vi "_Read.vi"(8 "error in (no error)":errorcluster, 11 "Wavelength Meter in":refnum<class "Wavelength Meter.lvclass">) -> (0 "error out":errorcluster, 2 "4 Data Points":dbl[](array[numeric]), 3 "Wavelength Meter out":refnum<class "Wavelength Meter.lvclass">)   [LabVIEW 2023, in "Wavelength Meter.lvclass"]
uses:
  Wavelength Meter.lvclass
  Wavelength Meter.lvclass/Wavelength Meter.ctl
  Utility Classes/Readable/Readable.lvclass
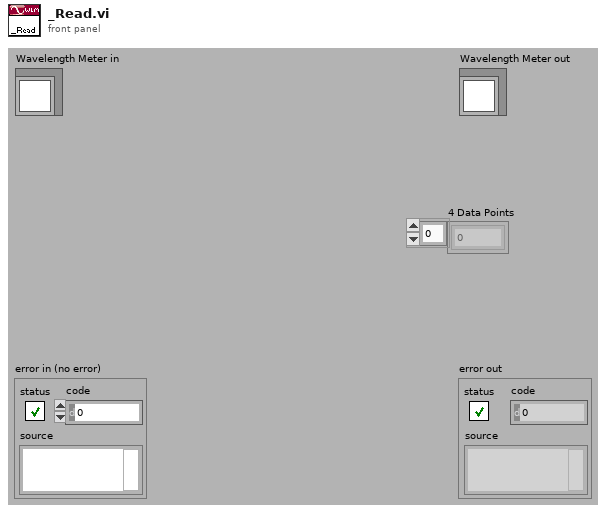
[diagram p1: front panel]
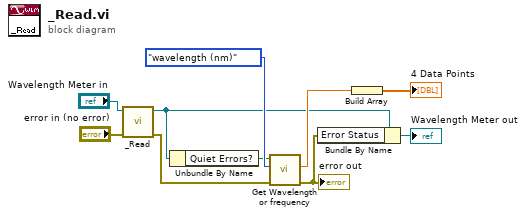
[diagram p0: block diagram]
diagram:
  n1 = call-parent "_Read.vi"("error in (no error)"="error in (no error)", "Readable in"="Wavelength Meter in") -> ("error out"=w5:errorcluster, "Readable out"=w4:refnum<class "Wavelength Meter.lvclass">)  [unwired: 8 out]
  n2 = Unbundle By Name(w4) -> ("Quiet Errors?"=w2:bool)
  n3 = call "Get Wavelength or frequency.vi"("error in (no error)"=w5, "mode (wavelength)"=enum16{"wavelength (nm)", "frequency (THz)"}."wavelength (nm)", "Quiet Errors?"=w2) -> ("error out"=w1:errorcluster, "result"=w7:dbl)  [unwired: 1 in, 6 out]
  "error out" <- w1
  n4 = Bundle By Name(cluster=w4, "Error Status"=w1) -> (→"Wavelength Meter out":refnum<class "Wavelength Meter.lvclass">)
  n5 = Build Array(w7) -> (→"4 Data Points":dbl[])
